vi "gyro pll async.vi"(11 "pll event pair":T8) -> ()   [LabVIEW 2020]
uses:
  PID action.ctl
  pll parameters.ctl
  PID - mode.ctl
  lorentzian.ctl
  circle corners.ctl
  pll talkback data type.ctl
  server talk-to-back pair.ctl
  server talkback message type.ctl
  server talkto message type.ctl
  pid -- parameters.ctl
  agregator -- action.ctl
  interpolation state - real.ctl
  data source action.ctl
  four-corner circle transformation.ctl
  publisher action.ctl
  linear interpolation - real.vi
  Q -- check range -- i -- real.vi
  linear interpolation iiii- complex.vi
  <vilib>/Analysis/baseanly.llb/A x B.vi
  <vilib>/Analysis/baseanly.llb/Complex A x B.vi
  line -- complex.vi
  Q -- check range -- i -- integer.vi
  Q - not nan -- real.vi
  Q - not nan -- integer.vi
  <vilib>/Analysis/Matrix/Numeric/Conversions/Array To Matrix.vi
  <vilib>/Analysis/Matrix/Numeric/Conversions/Array To Matrix - RA2.vi
  <vilib>/Analysis/baseanly.llb/Inverse Matrix.vi
  <vilib>/Analysis/baseanly.llb/Real Inverse Matrix.vi
panel:
  in  "main":enum32{"Page 1", "Page 2", "Page 3"}(tab)
  in  "pll parameters":T1={"PID mode"=enum."normal", "plot hist time (sec)"=1.0, "dt (sec)"=0.001, "visc hist time (sec)"=2.0, "time int ave time (sec)"=0.3, "PLL limits (Hz)"=5000.0} {"PLL limits (Hz)" format="%#.2f"; "time int ave time (sec)" format="%#_10f"; "visc hist time (sec)" format="%#_10f"; "dt (sec)" format="%#_10f"; "plot hist time (sec)" format="%#_10f"}
  in  "PID parameters :{}[];'":T3={"I (sec)"=0.004634123928756344, "P (sec)"=0.008980860327047186} {"P (sec)" scale=0.01..10.0; "I (sec)" scale=0.01..10.0}
  out "results":T4={"freq (Hz)"=40017.438097734725, "gamma (Hz)"=6.817921124952451, "Voltage (V)"=6.817921124952451+0.0i, "overlimit ?"=FALSE} {"Voltage (V)" format="%#.4f"; "gamma (Hz)" format="%#.4f"; "freq (Hz)" format="%#.11f"}
  out "PLL is ON ?":bool
  in  "Do reset frequency -- PID action":T5=enum."reset frequency"
  in  "Do reset frequency source":dbl=15.0 format="%#_10f"
  out "zi freq temporary":dbl=40015.59220124337 format="%#.2f"
  out "DO reset freq !":bool
  in  "lorentzian":T6={"A (VHz)"=1.0, "f (Hz)"=1000.0, "G (Hz)"=3.0, "phi(rad)"=0.0, "Q"=300.0, "Norm  Ampl"=nan, "bg (V)"=0.0+0.0i, "4corners"={"z (-pi/2)"=9.277908004825974e-07+0.0007240755403629966i, "z(inf)"=2.6527949823343002e-05+0.0007477540585896028i, "z (pi/2)"=2.8494315967368497e-06+0.0007733542176124632i, "z center"=1.8886111986097237e-06+0.0007487148789877299i, "z(0)"=-2.2750727426123552e-05+0.000749675699385857i, "radius"=2.4658065287076567e-05}} {"bg (V)" format="%#9_9f"; "Q" format="%#9_9f"; "phi(rad)" format="%#9_9f"; "G (Hz)" format="%#9_9f"; "f (Hz)" format="%#9_9f"}
  out "Stoped?":bool
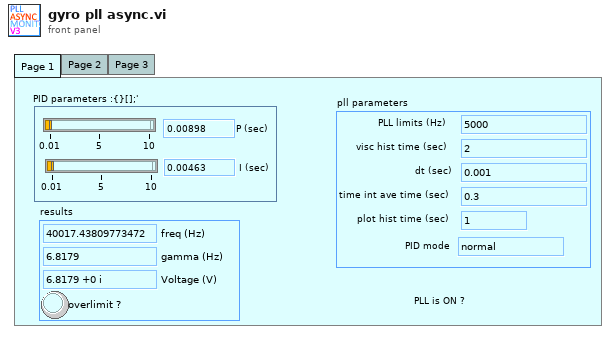
[diagram p1: front panel]
types:
  T1 = typedef "pll parameters.ctl" = cluster{"PID mode":T2, "plot hist time (sec)":dbl, "dt (sec)":dbl, "visc hist time (sec)":dbl, "time int ave time (sec)":dbl, "PLL limits (Hz)":dbl}
  T2 = typedef "PID - mode.ctl" = enum16{"normal", "heat"}
  T3 = typedef "pid -- parameters.ctl" = cluster{"I (sec)":dbl, "P (sec)":dbl}
  T4 = typedef "pll talkback data type.ctl" = cluster{"freq (Hz)":dbl, "gamma (Hz)":dbl, "Voltage (V)":cdb, "overlimit ?":bool}
  T5 = typedef "PID action.ctl" = enum16{"append", "empty!", "reset frequency", "reset from num", "overlimit"}
  T6 = typedef "lorentzian.ctl" = cluster{"A (VHz)":dbl, "f (Hz)":dbl, "G (Hz)":dbl, "phi(rad)":dbl, "Q":dbl, "Norm  Ampl":dbl, "bg (V)":cdb, "4corners":T7}
  T7 = typedef "circle corners.ctl" = cluster{"z (-pi/2)":cdb, "z(inf)":cdb, "z (pi/2)":cdb, "z center":cdb, "z(0)":cdb, "radius":dbl}
  T8 = typedef "server talk-to-back pair.ctl" = cluster{"talkback event":refnum<user-event>, "talkto event":refnum<user-event>}
  T9 = typedef "interpolation state - real.ctl" = cluster{"requested size":i32, "Array":dbl[], "actual number of elements":i32}
  T10 = typedef "agregator -- action.ctl" = enum16{"append", "interpolate", "empty!", "force", "init", "scale", "read last"}
  T11 = typedef "server talkback message type.ctl" = cluster{"message":enum16{"new", "void"}}
  T12 = typedef "publisher action.ctl" = enum16{"set", "get", "init", "check"}
  T13 = typedef "data source action.ctl" = enum16{"set", "get", "init", "set-and-get", "init source"}
  T14 = typedef "four-corner circle transformation.ctl" = enum16{"z(c) z(inf)", "z(c) z(zero)", "fix phase", "calculate lorentzian", "z(0) z(+-pi/2)", "shift to zcenter", "to  canonical", "get canonical phase", "get4corners", "update lorentzian -- from z0", "fake gamma normal", "fake gamma heat", "calculate complex slope"}
  T15 = typedef "PLL data source.ctl" = enum16{"meta", "MFLI", "SRS865A", "arydh"}
  T16 = typedef "interpolation state - complex.ctl" = cluster{"requested size":i32, "Array":cdb[], "actual number of elements":i32}
  T17 = typedef "eventvkey.ctl" = enum16{"ASCII", "Enter", "Return", "Shift", "Ctrl", "Alt", "Cmd", "Opt", "Caps", "NumLock", "Clear", "Break", "Up", "Down", "Left", "Right", "Insert", "Delete", "Home", "End", "PageUp", "PageDown", "Escape", "Help", "Pause", "ScrollLock", "F1", "F2", "F3", "F4", "F5", "F6", "F7", "F8", "F9", "F10", "F11", "F12", "F13", "F14", "F15", "F16", "F17", "F18", "F19", "F20", "F21", "F22", "F23", "F24", "Play", "VolumeUp", "VolumeDown", "Mute", "Two Byte Char"}
  T18 = enum16{"stop", "start", "update pars", "update request", "new", "launch", "exit", "get", "reset", "pause", "unpause"}
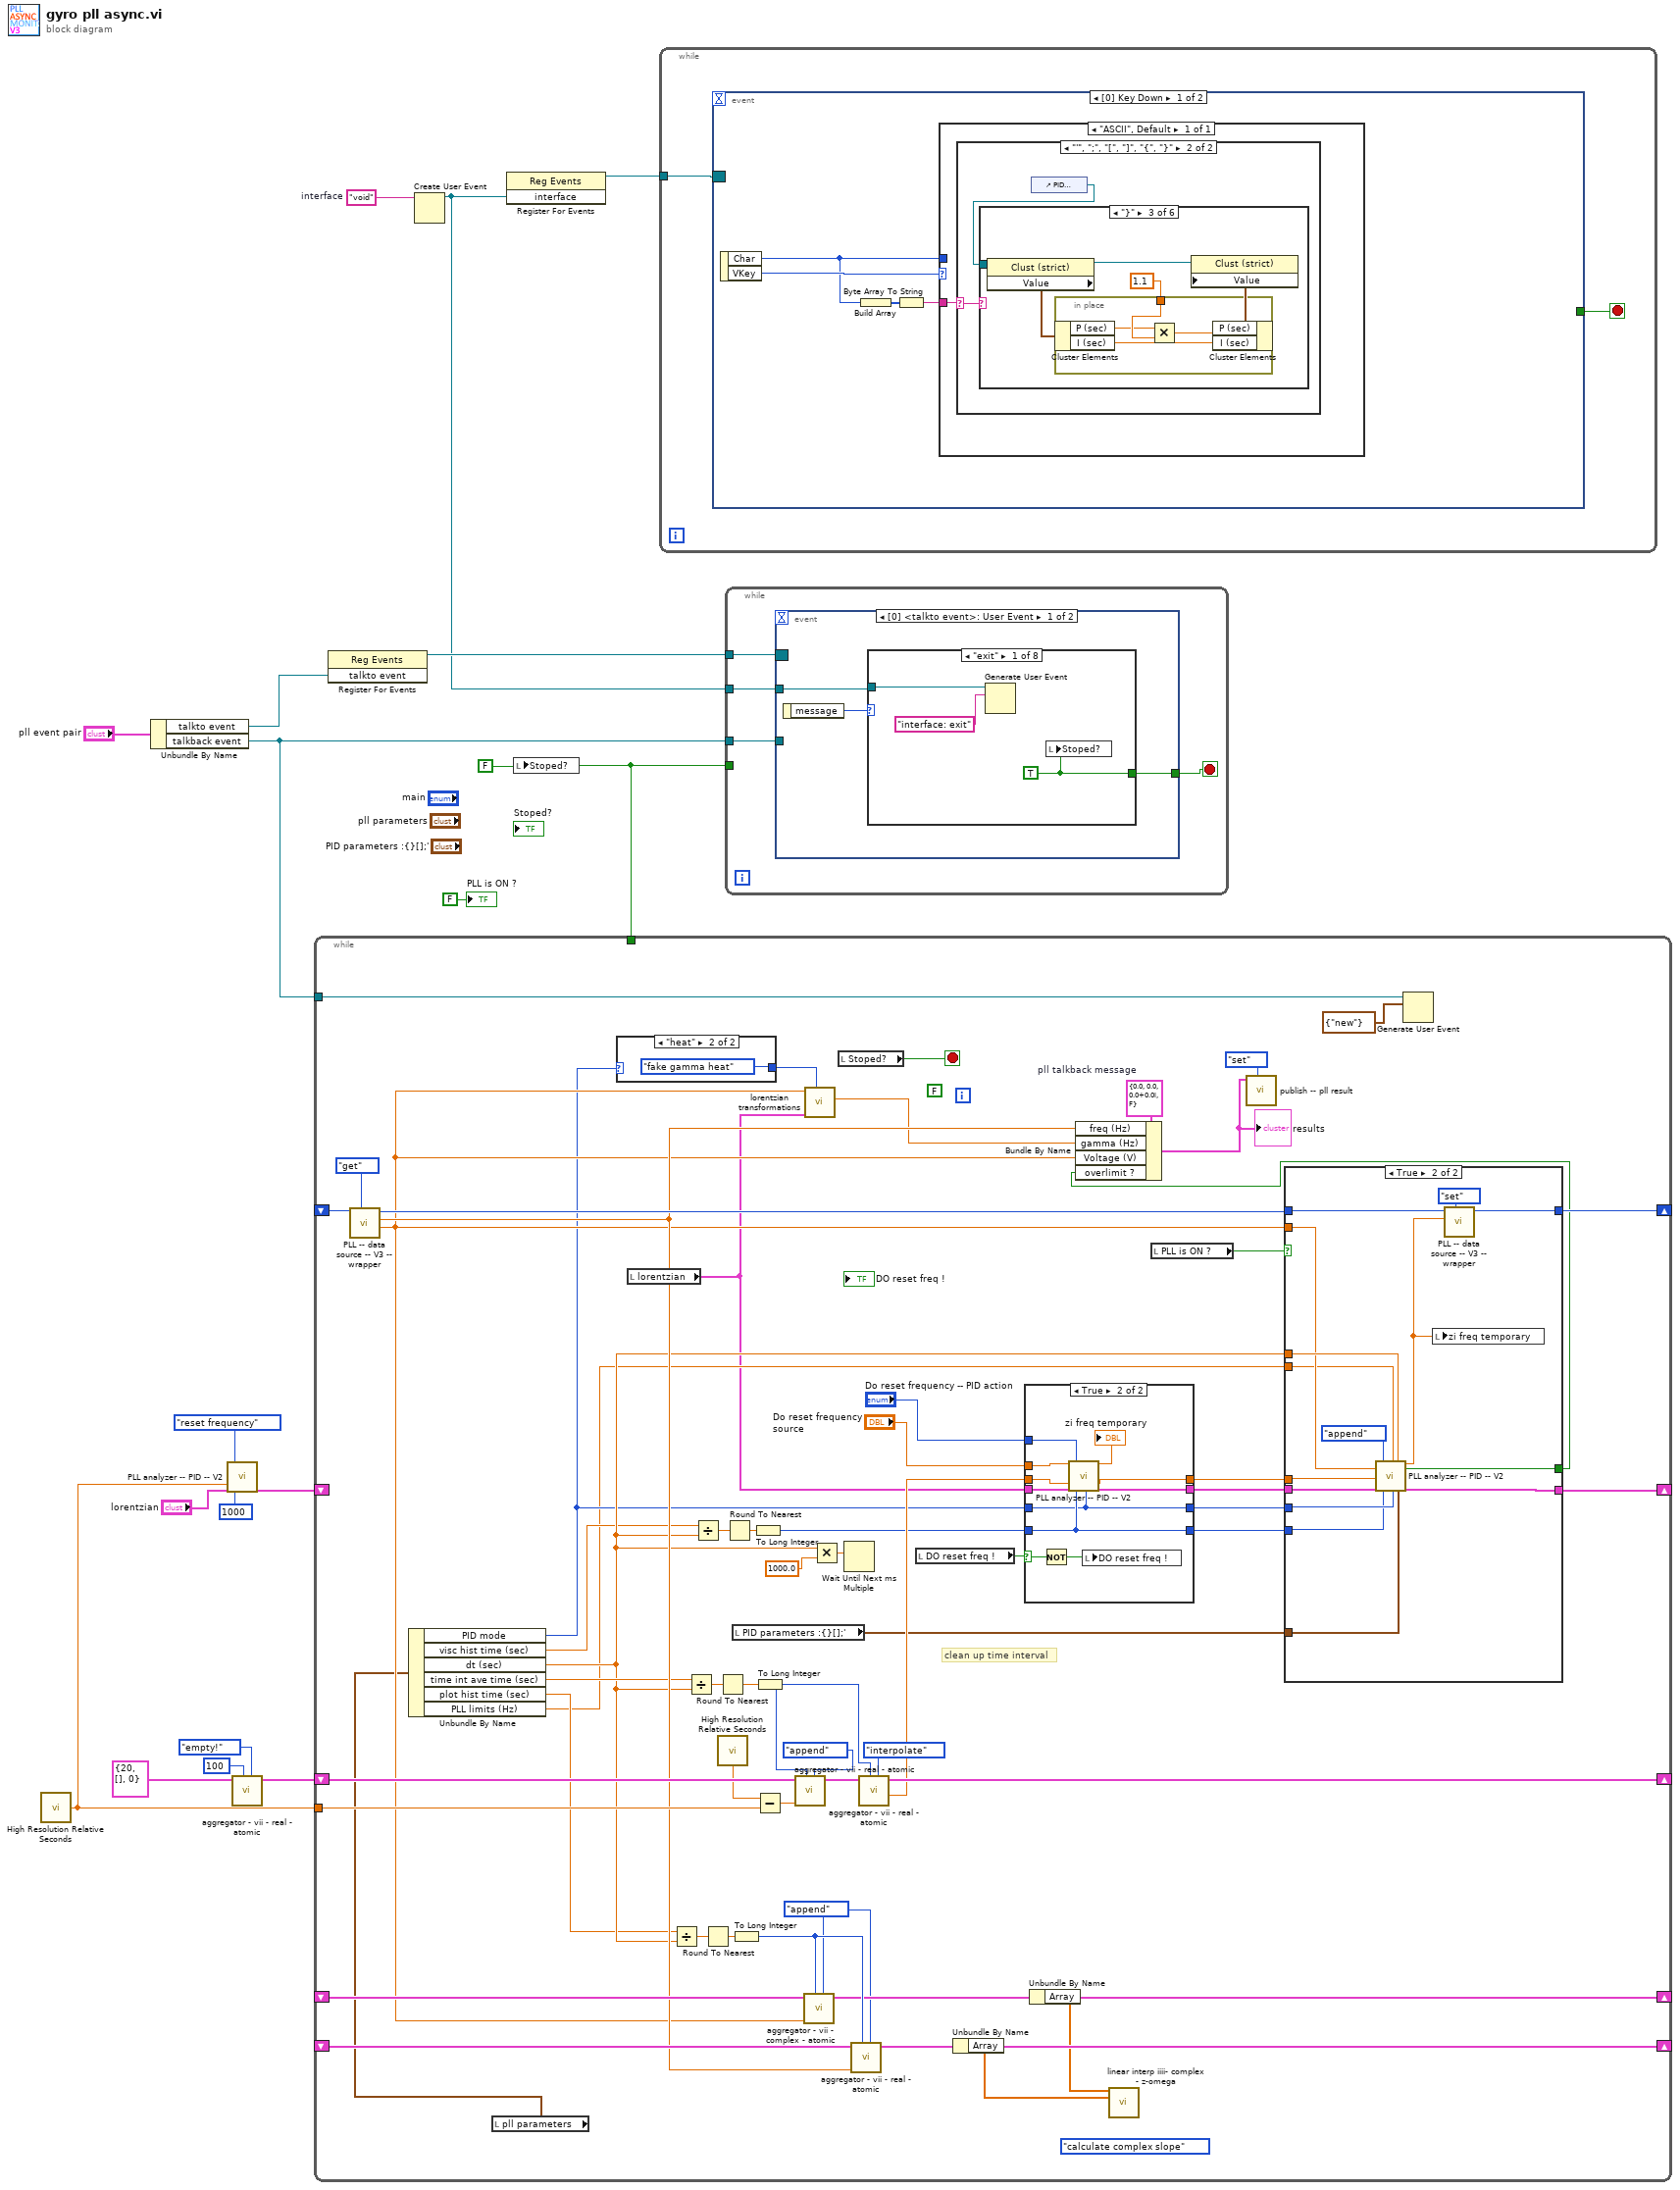
[diagram p0: block diagram]
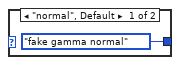
[diagram p2: hidden frame]
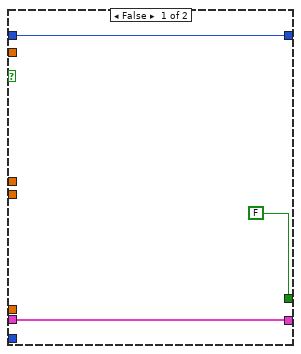
[diagram p3: hidden frame]
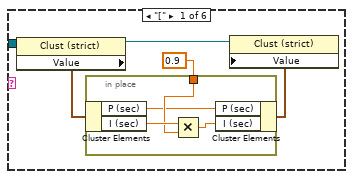
[diagram p6: hidden frame]
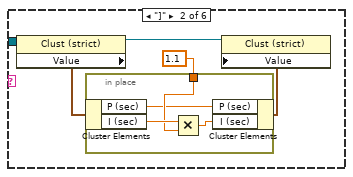
[diagram p7: hidden frame]
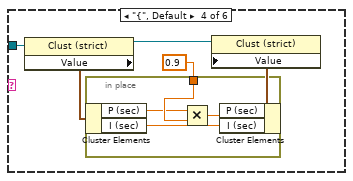
[diagram p8: hidden frame]
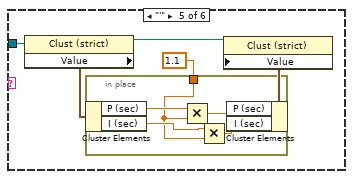
[diagram p9: hidden frame]
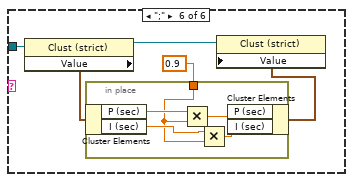
[diagram p10: hidden frame]
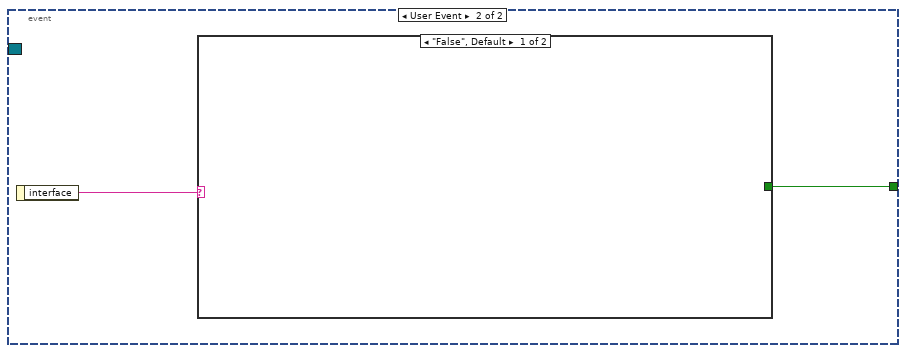
[diagram p11: hidden frame]
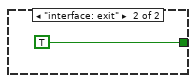
[diagram p12: hidden frame]
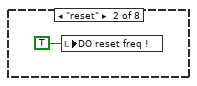
[diagram p13: hidden frame]
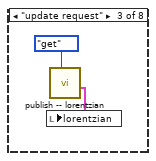
[diagram p14: hidden frame]
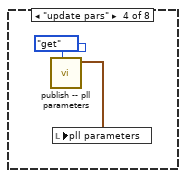
[diagram p15: hidden frame]
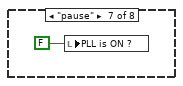
[diagram p18: hidden frame]
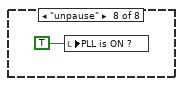
[diagram p19: hidden frame]
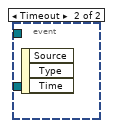
[diagram p20: hidden frame]
diagram:
  w3 = "void"  # interface
  w4 = FALSE ("Stop")
  n1 = call <vilib>:"High Resolution Relative Seconds.vi"() -> ("relative seconds"=w6:dbl)
  n2 = Unbundle By Name("pll event pair") -> ("talkto event"=w14:refnum<user-event>, "talkback event"=w15:refnum<user-event>)
  n3 = call "PLL analyzer -- PID -- V2.vi"("time in (sec)"=w6, "lorentzian IN"="lorentzian", "PID action"=PID_action."reset frequency", "requested size"=1000) -> ("lorentzian  OUT"=w9:T6)  [unwired: 12 in, 3 out]
  n4 = call "aggregator - vii - real - atomic.vi"("aggregator action"=agregator_--_action."empty!", "requested size"=100, "state IN"=T9 {"requested size"=20, "Array"=[], "actual number of elements"=0}) -> ("state OUT"=w12:T9)  [unwired: 5 in, 3 out]
  n5 = while {
    tunnel: w6 -> [w78]
    shift-right: [w76] -> _
    shift-left: w9 -> [_]
    shift-right: [w44] -> _
    shift-left: _ -> [w75]
    shift-right: [w73] -> _
    shift-left: _ -> [w74]
    shift-right: [w68] -> _
    shift-left: w12 -> [w71]
    shift-right: [w63] -> _
    shift-left: _ -> [w59]
    tunnel: w15 -> [w21]
    tunnel: w4 -> [_]
    stop <- w24 stop-if-true
    (unwired) FALSE
    w36 = T4 {"freq (Hz)"=0.0, "gamma (Hz)"=0.0, "Voltage (V)"=0.0+0.0i, "overlimit ?"=FALSE}  # pll talkback message
    (unwired) four-corner_circle_transformation."calculate complex slope" ("4 corner circle transformation")
    w19 = agregator_--_action."append" ("aggregator action")
    # "clean up time interval"
    n6 = call "PLL -- data source -- V3 -- wrapper.vi"("data source action"=data_source_action."get", "PLL data source"=w59) -> ("z out (V)"=w39:cdb, "Freq out (Hz)"=w43:dbl, "PLL data source OUT"=w61:T15)  [unwired: 7 in]
    n7 = local read "pll parameters"() -> (w31:T1)
    n8 = Unbundle By Name(w31) -> ("PID mode"=w32:T2, "visc hist time (sec)"=w33:dbl, "dt (sec)"=w34:dbl, "time int ave time (sec)"=w35:dbl, "plot hist time (sec)"=w30:dbl, "PLL limits (Hz)"=w28:dbl)
    n9 = case shown="\"heat\"" w32 {
      tunnel: [four-corner_circle_transformation."fake gamma normal" ("4 corner circle transformation") four-corner_circle_transformation."fake gamma heat" ("4 corner circle transformation")] -> w41
      frame "normal", Default {
      }
      frame "heat" {
      }
    }
    n10 = local read "lorentzian"() -> (w25:T6)
    n11 = Divide(x=w30, y=w34) -> (x/y=w48:dbl)
    n12 = Divide(x=w35, y=w34) -> (x/y=w52:dbl)
    n13 = Divide(x=w33, y=w34) -> (x/y=w55:dbl)
    n14 = Round To Nearest(number=w48) -> (nearest integer value=w47:dbl)
    n15 = Round To Nearest(number=w52) -> (nearest integer value=w51:dbl)
    n16 = call <vilib>:"High Resolution Relative Seconds.vi"() -> ("relative seconds"=w62:dbl)
    n17 = Round To Nearest(number=w55) -> (nearest integer value=w54:dbl)
    n18 = To Long Integer(number=w47) -> (32bit integer=w46:i32)
    n19 = local read "PID parameters :{}[];'"() -> (w22:T3)
    n20 = To Long Integer(number=w54) -> (32bit integer=w53:i32)
    n21 = To Long Integer(number=w51) -> (32bit integer=w50:i32)
    n22 = Subtract(x=w62, y=w78) -> (x-y=w70:dbl)
    n23 = call "aggregator - vii - real - atomic.vi"("aggregator action"=agregator_--_action."append", "requested size"=w50, "number"=w70, "state IN"=w71) -> ("state OUT"=w69:T9)  [unwired: 4 in, 3 out]
    n24 = call "aggregator - vii - complex - atomic.vi"("aggregator action"=w19, "requested size"=w46, "number"=w39, "state IN"=w75) -> ("state OUT"=w44:T16)  [unwired: 4 in, 3 out]
    n25 = call "lorentzian transformations.vi"("4 corner circle transformation"=w41, "lorentzian in"=w25, "voltage in"=w39) -> ("gamma OUT"=w40:dbl)  [unwired: 5 in, 3 out]
    n26 = Multiply(x=w34, y=1000.0) -> (x*y=w66:dbl)
    n27 = local read "Stoped?"() -> (w24:bool)
    n28 = Wait Until Next ms Multiple(millisecond multiple=w66) -> ()  [unwired: 1 out]
    n29 = call "aggregator - vii - real - atomic.vi"("aggregator action"=w19, "requested size"=w46, "number"=w43, "state IN"=w74) -> ("state OUT"=w73:T9)  [unwired: 4 in, 3 out]
    n30 = call "aggregator - vii - real - atomic.vi"("aggregator action"=agregator_--_action."interpolate", "requested size"=w50, "state IN"=w69) -> ("interp average"=w57:dbl, "state OUT"=w68:T9)  [unwired: 5 in, 2 out]
    n31 = local read "DO reset freq !"() -> (w65:bool)
    n32 = Unbundle By Name(w73) -> ("Array"=w37:dbl[])
    n33 = case shown="True" w65 {
      selector: w65 -> [_ w111]
      tunnel: w25 -> [w102 w113]
      tunnel: [w102 w112] -> w64
      tunnel: w53 -> [w101 w108]
      tunnel: [w101 w108] -> w58
      tunnel: w57 -> [w100 w107]
      tunnel: "Do reset frequency -- PID action" -> [_ w106]
      tunnel: "Do reset frequency source" -> [_ w105]
      tunnel: [w100 w104] -> w49
      tunnel: w32 -> [w99 w103]
      tunnel: [w99 w103] -> w45
      frame False {
      }
      frame True {
        n34 = Not(x=w111) -> (.not. x?=w110:bool)
        n35 = call "PLL analyzer -- PID -- V2.vi"("frequency IN (Hz)"=w105, "time in (sec)"=w107, "lorentzian IN"=w113, "PID action"=w106, "requested size"=w108, "PID mode"=w103) -> ("frequency OUT (Hz)"=→"zi freq temporary":dbl, "time out (sec)"=w104:dbl, "lorentzian  OUT"=w112:T6)  [unwired: 10 in, 1 out]
        n36 = local write "DO reset freq !"(w110) -> ()
      }
    }
    n37 = Unbundle By Name(w44) -> ("Array"=w38:cdb[])
    n38 = call "linear interp iiii- complex - z-omega.vi"("z"=w38, "omega"=w37) -> ()  [unwired: 5 in, 9 out]
    n39 = local read "PLL is ON ?"() -> (w23:bool)
    n40 = case shown="True" w23 {
      tunnel: [w83 w98] -> w76
      tunnel: w58 -> [_ w89]
      tunnel: w39 -> [_ w87]
      tunnel: w49 -> [_ w93]
      tunnel: w64 -> [w83 w90]
      tunnel: [w82 w96] -> w63
      tunnel: w61 -> [w82 w94]
      tunnel: w34 -> [_ w92]
      tunnel: w45 -> [_ w91]
      tunnel: w22 -> [_ w86]
      tunnel: [FALSE w85] -> w29
      tunnel: w28 -> [_ w84]
      frame False {
      }
      frame True {
        n41 = call "PLL analyzer -- PID -- V2.vi"("voltage IN (V)"=w87, "time in (sec)"=w93, "lorentzian IN"=w90, "PID action"=PID_action."append", "requested size"=w89, "PLL limits (Hz)"=w84, "PID mode"=w91, "dt (sec)"=w92, "PID parameters"=w86) -> ("frequency OUT (Hz)"=w88:dbl, "overlimit ?"=w85:bool, "lorentzian  OUT"=w98:T6)  [unwired: 7 in, 1 out]
        n42 = local write "zi freq temporary"(w88) -> ()
        n43 = call "PLL -- data source -- V3 -- wrapper.vi"("data source action"=data_source_action."set", "Freq in (Hz)"=w88, "PLL data source"=w94) -> ("PLL data source OUT"=w96:T15)  [unwired: 6 in, 2 out]
      }
    }
    n44 = Bundle By Name(cluster=w36, "freq (Hz)"=w43, "gamma (Hz)"=w40, "Voltage (V)"=w39, "overlimit ?"=w29) -> (w27:T4)
    "results" <- w27
    n45 = call "publish -- pll result.vi"("publisher action"=publisher_action."set", "pll result IN"=w27) -> ()  [unwired: 9 in, 1 out]
    n46 = Generate User Event(user event=w21, event data cluster=T11 {"message"=enum."new"} ("event data")) -> ()  [unwired: 2 in, 2 out]
  }
  n47 = register-events(w14) -> (reference out=w18:refnum<event-registration>)  [unwired: 2 in, 1 out]
  n48 = Create User Event(user event datatype=w3) -> (user event=w1:refnum<user-event>)  [unwired: 1 in, 1 out]
  n49 = register-events(w1) -> (reference out=w2:refnum<event-registration>)  [unwired: 2 in, 1 out]
  n50 = local write "Stoped?"(w4) -> ()
  n51 = while {
    tunnel: w2 -> [w115]
    stop <- w114 stop-if-true
    n52 = event shown="[0] Key Down" {
      selector: w115 -> [_ _]
      dyn-events: _ -> [_ _]
      timeout: _ -> [_ _]
      tunnel: [_ w179] -> w114
      event Key Down {
        n53 = event-data() -> ("Char"=w117:i16, "VKey"=w119:T17)  [unwired: 1 in]
        n54 = Build Array(w117) -> (w118:i16[])
        n55 = Byte Array To String(unsigned byte array=w118) -> (string=w116:string)
        n56 = case shown="\"ASCII\", Default" w119 {
          tunnel: w117 -> [_]
          tunnel: w116 -> [w120]
          frame "ASCII", Default {
            n57 = case shown="\"'\", \";\", \"[\", \"]\", \"{\", \"}\"" w120 {
              selector: w120 -> [_ w122]
              frame "0", Default {
              }
              frame "'", ";", "[", "]", "{", "}" {
                n58 = control-ref of="PID parameters :{}[];'"() -> (w121:refnum<vi>)
                n59 = case shown="\"}\"" w122 {
                  tunnel: w121 -> [w127 w136 w145 w154 w163 w173]
                  frame "[" {
                    n60 = property class="Clust (strict)"(reference=w127) -> (reference out=w126:refnum<vi>, "Value"=w125:T3)  [unwired: 1 in, 1 out]
                    n61 = in-place {
                      in-place-border: 0.9 -> [w130]
                      n62 = in-place-cluster #1(w125) -> ("P (sec)"=w128:dbl, "I (sec)"=w131:dbl)
                      n63 = Multiply(x=w131, y=w130) -> (x*y=w129:dbl)
                      n64 = in-place-cluster #1("P (sec)"=w128, "I (sec)"=w129) -> (w124:T3)
                    }
                    n65 = property class="Clust (strict)"(reference=w126, "Value"=w124) -> ()  [unwired: 1 in, 2 out]
                  }
                  frame "]" {
                    n66 = property class="Clust (strict)"(reference=w136) -> (reference out=w135:refnum<vi>, "Value"=w134:T3)  [unwired: 1 in, 1 out]
                    n67 = in-place {
                      in-place-border: 1.1 -> [w139]
                      n68 = in-place-cluster #2(w134) -> ("P (sec)"=w137:dbl, "I (sec)"=w140:dbl)
                      n69 = Multiply(x=w140, y=w139) -> (x*y=w138:dbl)
                      n70 = in-place-cluster #2("P (sec)"=w137, "I (sec)"=w138) -> (w133:T3)
                    }
                    n71 = property class="Clust (strict)"(reference=w135, "Value"=w133) -> ()  [unwired: 1 in, 2 out]
                  }
                  frame "}" {
                    n72 = property class="Clust (strict)"(reference=w145) -> (reference out=w144:refnum<vi>, "Value"=w143:T3)  [unwired: 1 in, 1 out]
                    n73 = in-place {
                      in-place-border: 1.1 -> [w149]
                      n74 = in-place-cluster #3(w143) -> ("P (sec)"=w148:dbl, "I (sec)"=w146:dbl)
                      n75 = Multiply(x=w148, y=w149) -> (x*y=w147:dbl)
                      n76 = in-place-cluster #3("P (sec)"=w147, "I (sec)"=w146) -> (w142:T3)
                    }
                    n77 = property class="Clust (strict)"(reference=w144, "Value"=w142) -> ()  [unwired: 1 in, 2 out]
                  }
                  frame "{", Default {
                    n78 = property class="Clust (strict)"(reference=w154) -> (reference out=w153:refnum<vi>, "Value"=w152:T3)  [unwired: 1 in, 1 out]
                    n79 = in-place {
                      in-place-border: 0.9 -> [w158]
                      n80 = in-place-cluster #4(w152) -> ("P (sec)"=w157:dbl, "I (sec)"=w155:dbl)
                      n81 = Multiply(x=w157, y=w158) -> (x*y=w156:dbl)
                      n82 = in-place-cluster #4("P (sec)"=w156, "I (sec)"=w155) -> (w151:T3)
                    }
                    n83 = property class="Clust (strict)"(reference=w153, "Value"=w151) -> ()  [unwired: 1 in, 2 out]
                  }
                  frame "'" {
                    n84 = property class="Clust (strict)"(reference=w163) -> (reference out=w162:refnum<vi>, "Value"=w161:T3)  [unwired: 1 in, 1 out]
                    n85 = in-place {
                      in-place-border: 1.1 -> [w164]
                      n86 = in-place-cluster #5(w161) -> ("P (sec)"=w168:dbl, "I (sec)"=w166:dbl)
                      n87 = Multiply(x=w168, y=w164) -> (x*y=w167:dbl)
                      n88 = Multiply(x=w166, y=w164) -> (x*y=w165:dbl)
                      n89 = in-place-cluster #5("P (sec)"=w167, "I (sec)"=w165) -> (w160:T3)
                    }
                    n90 = property class="Clust (strict)"(reference=w162, "Value"=w160) -> ()  [unwired: 1 in, 2 out]
                  }
                  frame ";" {
                    n91 = property class="Clust (strict)"(reference=w173) -> (reference out=w172:refnum<vi>, "Value"=w171:T3)  [unwired: 1 in, 1 out]
                    n92 = in-place {
                      in-place-border: 0.9 -> [w174]
                      n93 = in-place-cluster #6(w171) -> ("P (sec)"=w178:dbl, "I (sec)"=w176:dbl)
                      n94 = Multiply(x=w178, y=w174) -> (x*y=w177:dbl)
                      n95 = Multiply(x=w176, y=w174) -> (x*y=w175:dbl)
                      n96 = in-place-cluster #6("P (sec)"=w177, "I (sec)"=w175) -> (w170:T3)
                    }
                    n97 = property class="Clust (strict)"(reference=w172, "Value"=w170) -> ()  [unwired: 1 in, 2 out]
                  }
                }
              }
            }
          }
        }
      }
      event User Event {
        n98 = event-data() -> ("interface"=w180:string)  [unwired: 1 in]
        n99 = case shown="\"False\", Default" w180 {
          tunnel: [_ TRUE] -> w179
          frame "False", Default {
          }
          frame "interface: exit" {
          }
        }
      }
    }
  }
  n100 = while {
    tunnel: w18 -> [w185]
    tunnel: w15 -> [w184]
    tunnel: w4 -> [_]
    tunnel: w1 -> [w182]
    stop <- w183 stop-if-true
    n101 = event shown="[0] <talkto event>: User Event" {
      selector: w185 -> [_ _]
      dyn-events: _ -> [_ _]
      timeout: _ -> [_ _]
      tunnel: w184 -> [_ _]
      tunnel: [w187 _] -> w183
      tunnel: w182 -> [w186 _]
      event User Event {
        n102 = event-data() -> ("message"=w188:T18)  [unwired: 1 in]
        n103 = case shown="\"exit\"" w188 {
          tunnel: [w191 _ _ _ _ _ _ _] -> w187
          tunnel: w186 -> [w190 _ _ _ _ _ _ _]
          frame "exit" {
            w191 = TRUE
            n104 = Generate User Event(user event=w190, event data cluster="interface: exit" ("event data")) -> ()  [unwired: 2 in, 2 out]
            n105 = local write "Stoped?"(w191) -> ()
          }
          frame "reset" {
            n106 = local write "DO reset freq !"(TRUE) -> ()
          }
          frame "update request" {
            n107 = call "publish -- lorentzian.vi"("publisher action"=publisher_action."get") -> ("lorentzian OUT"=w193:T6)  [unwired: 10 in]
            n108 = local write "lorentzian"(w193) -> ()
          }
          frame "update pars" {
            n109 = call "publish -- pll parameters.vi"("publisher action"=publisher_action."get") -> ("pll parameters OUT"=w195:T1)  [unwired: 10 in]
            n110 = local write "pll parameters"(w195) -> ()
          }
          frame "start", Default {
          }
          frame "stop" {
          }
          frame "pause" {
            n111 = local write "PLL is ON ?"(FALSE ("Stoped?")) -> ()
          }
          frame "unpause" {
            n112 = local write "PLL is ON ?"(TRUE ("Stoped?")) -> ()
          }
        }
      }
      event Timeout {
        n113 = event-data() -> ()  [unwired: 1 in, 3 out]
      }
    }
  }
  "PLL is ON ?" <- FALSE ("unpaused?")
